vi "SwapXY.vi"(11 "Point":cluster{"X Cen":sgl, "Y Cen":sgl}={"X Cen"=500.0, "Y Cen"=500.0}) -> (3 "Swapped":cluster{"X Cen":sgl, "Y Cen":sgl}={"X Cen"=500.0, "Y Cen"=500.0})   [LabVIEW 2014]
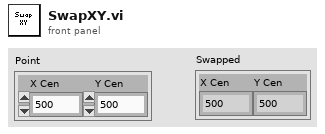
[diagram p1: front panel]
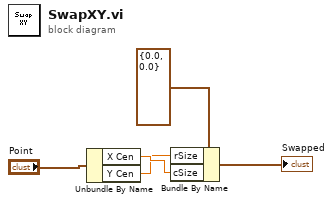
[diagram p0: block diagram]
diagram:
  n1 = Unbundle By Name("Point") -> ("X Cen"=w5:sgl, "Y Cen"=w4:sgl)
  n2 = Bundle By Name(cluster=cluster{"rSize":sgl, "cSize":sgl} {"rSize"=0.0, "cSize"=0.0} ("WindowSize"), "rSize"=w4, "cSize"=w5) -> (→"Swapped":cluster{"rSize":sgl, "cSize":sgl})
